vi "RTS Set Chamber Temp Humidity.vi"(5 "Room Setpoints":T7={"Room Setpoint Temperature (*RM Dry Set P1)"=90.0, "Room Setpoint Humidity (*RM Hum Set P1)"=20.0, "Room Cool Temperature (*RM Cool Setp 1)"=65.0, "Room Dehum Temperature (*RM De Hum Set P1)"=60.0} {"Room Dehum Temperature (*RM De Hum Set P1)" min=30.0 max=120.0; "Room Cool Temperature (*RM Cool Setp 1)" min=30.0 max=120.0; "Room Setpoint Humidity (*RM Hum Set P1)" min=5.0 max=98.0; "Room Setpoint Temperature (*RM Dry Set P1)" min=40.0 max=120.0}, 7 "All Door Opener Ctrl":T4 {"Station 8"."Station Slide"."Chamber 1-1"."Start Time" format="%<%X\n%x>T"; "Station 8"."Station Slide"."Chamber 1-1"."End Time" format="%<%X\n%x>T"; "Station 8"."Station Slide"."Time Count (s)" format="%.2f"; "Station 8"."Station Cab"."Chamber 1-1"."Start Time" format="%<%X\n%x>T"; "Station 8"."Station Cab"."Chamber 1-1"."End Time" format="%<%X\n%x>T"; "Station 8"."Station Cab"."Time Count (s)" format="%.2f"; "Station 8"."Station Freezer"."Chamber 1-1"."Start Time" format="%<%X\n%x>T"; "Station 8"."Station Freezer"."Chamber 1-1"."End Time" format="%<%X\n%x>T"; "Station 8"."Station Freezer"."Time Count (s)" format="%.2f"; "Station 7"."Station Slide"."Chamber 1-1"."Start Time" format="%<%X\n%x>T"; "Station 7"."Station Slide"."Chamber 1-1"."End Time" format="%<%X\n%x>T"; "Station 7"."Station Slide"."Time Count (s)" format="%.2f"; "Station 7"."Station Cab"."Chamber 1-1"."Start Time" format="%<%X\n%x>T"; "Station 7"."Station Cab"."Chamber 1-1"."End Time" format="%<%X\n%x>T"; "Station 7"."Station Cab"."Time Count (s)" format="%.2f"; "Station 7"."Station Freezer"."Chamber 1-1"."Start Time" format="%<%X\n%x>T"; "Station 7"."Station Freezer"."Chamber 1-1"."End Time" format="%<%X\n%x>T"; "Station 7"."Station Freezer"."Time Count (s)" format="%.2f"; "Station 6"."Station Slide"."Chamber 1-1"."Start Time" format="%<%X\n%x>T"; "Station 6"."Station Slide"."Chamber 1-1"."End Time" format="%<%X\n%x>T"; "Station 6"."Station Slide"."Time Count (s)" format="%.2f"; "Station 6"."Station Cab"."Chamber 1-1"."Start Time" format="%<%X\n%x>T"; "Station 6"."Station Cab"."Chamber 1-1"."End Time" format="%<%X\n%x>T"; "Station 6"."Station Cab"."Time Count (s)" format="%.2f"; "Station 6"."Station Freezer"."Chamber 1-1"."Start Time" format="%<%X\n%x>T"; "Station 6"."Station Freezer"."Chamber 1-1"."End Time" format="%<%X\n%x>T"; "Station 6"."Station Freezer"."Time Count (s)" format="%.2f"; "Station 5"."Station Slide"."Chamber 1-1"."Start Time" format="%<%X\n%x>T"; "Station 5"."Station Slide"."Chamber 1-1"."End Time" format="%<%X\n%x>T"; "Station 5"."Station Slide"."Time Count (s)" format="%.2f"; "Station 5"."Station Cab"."Chamber 1-1"."Start Time" format="%<%X\n%x>T"; "Station 5"."Station Cab"."Chamber 1-1"."End Time" format="%<%X\n%x>T"; "Station 5"."Station Cab"."Time Count (s)" format="%.2f"; "Station 5"."Station Freezer"."Chamber 1-1"."Start Time" format="%<%X\n%x>T"; "Station 5"."Station Freezer"."Chamber 1-1"."End Time" format="%<%X\n%x>T"; "Station 5"."Station Freezer"."Time Count (s)" format="%.2f"; "Station 4"."Station Slide"."Chamber 1-1"."Start Time" format="%<%X\n%x>T"; "Station 4"."Station Slide"."Chamber 1-1"."End Time" format="%<%X\n%x>T"; "Station 4"."Station Slide"."Time Count (s)" format="%.2f"; "Station 4"."Station Cab"."Chamber 1-1"."Start Time" format="%<%X\n%x>T"; "Station 4"."Station Cab"."Chamber 1-1"."End Time" format="%<%X\n%x>T"; "Station 4"."Station Cab"."Time Count (s)" format="%.2f"; "Station 4"."Station Freezer"."Chamber 1-1"."Start Time" format="%<%X\n%x>T"; "Station 4"."Station Freezer"."Chamber 1-1"."End Time" format="%<%X\n%x>T"; "Station 4"."Station Freezer"."Time Count (s)" format="%.2f"; "Station 3"."Station Slide"."Chamber 1-1"."Start Time" format="%<%X\n%x>T"; "Station 3"."Station Slide"."Chamber 1-1"."End Time" format="%<%X\n%x>T"; "Station 3"."Station Slide"."Time Count (s)" format="%.2f"; "Station 3"."Station Cab"."Chamber 1-1"."Start Time" format="%<%X\n%x>T"; "Station 3"."Station Cab"."Chamber 1-1"."End Time" format="%<%X\n%x>T"; "Station 3"."Station Cab"."Time Count (s)" format="%.2f"; "Station 3"."Station Freezer"."Chamber 1-1"."Start Time" format="%<%X\n%x>T"; "Station 3"."Station Freezer"."Chamber 1-1"."End Time" format="%<%X\n%x>T"; "Station 3"."Station Freezer"."Time Count (s)" format="%.2f"; "Station 2"."Station Slide"."Chamber 1-1"."Start Time" format="%<%X\n%x>T"; "Station 2"."Station Slide"."Chamber 1-1"."End Time" format="%<%X\n%x>T"; "Station 2"."Station Slide"."Time Count (s)" format="%.2f"; "Station 2"."Station Cab"."Chamber 1-1"."Start Time" format="%<%X\n%x>T"; "Station 2"."Station Cab"."Chamber 1-1"."End Time" format="%<%X\n%x>T"; "Station 2"."Station Cab"."Time Count (s)" format="%.2f"; "Station 2"."Station Freezer"."Chamber 1-1"."Start Time" format="%<%X\n%x>T"; "Station 2"."Station Freezer"."Chamber 1-1"."End Time" format="%<%X\n%x>T"; "Station 2"."Station Freezer"."Time Count (s)" format="%.2f"; "Station 1"."Station Slide"."Chamber 1-1"."Start Time" format="%<%X\n%x>T"; "Station 1"."Station Slide"."Chamber 1-1"."End Time" format="%<%X\n%x>T"; "Station 1"."Station Slide"."Time Count (s)" format="%.2f"; "Station 1"."Station Cab"."Chamber 1-1"."Start Time" format="%<%X\n%x>T"; "Station 1"."Station Cab"."Chamber 1-1"."End Time" format="%<%X\n%x>T"; "Station 1"."Station Cab"."Time Count (s)" format="%.2f"; "Station 1"."Station Freezer"."Chamber 1-1"."Start Time" format="%<%X\n%x>T"; "Station 1"."Station Freezer"."Chamber 1-1"."End Time" format="%<%X\n%x>T"; "Station 1"."Station Freezer"."Time Count (s)" format="%.2f"}, 8 "Error In":errorcluster, 11 "Modbus Master in":refnum<class "Modbus Master.lvclass">) -> (0 "Error Out":errorcluster, 1 "Matching Setpoints?":bool, 2 "Set Chamber Conditions":bool, 3 "Modbus master out":refnum<class "Modbus Master.lvclass">, 4 "Chamber 1-1":T1 {"Start Time" format="%<%X\n%x>T"; "End Time" format="%<%X\n%x>T"}, 6 "Index":i32)   [LabVIEW 2016]
uses:
  Type Definitions/RTS Chamber Temperature Humidity Control.ctl
  <vilib>/NI/Modbus Library/API/Master/Modbus Master.lvclass
  Type Definitions/RTS All Station Door Opener Ctrl.ctl
  Type Definitions/RTS Station Relay Ops.ctl
  Type Definitions/RTS Door Opener Indicator.ctl
  Type Definitions/RTS Door Ops Client.ctl
  Type Definitions/RTS Door Opening Schedule.ctl
  Type Definitions/RTS Door Ops Sequence.ctl
panel:
  # "Chamber Conditions:"
  # "Chamber Conditions:"
  # "Chamber Conditions:"
  # "Chamber Conditions:"
  # "Chamber Conditions:"
  # "Chamber Conditions:"
  # "Chamber Conditions:"
  # "Chamber Conditions:"
  # "Chamber Conditions:"
  # "Chamber Conditions:"
  # "Chamber Conditions:"
  # "Chamber Conditions:"
  # "Chamber Conditions:"
  # "Chamber Conditions:"
  # "Chamber Conditions:"
  # "Chamber Conditions:"
  # "Chamber Conditions:"
  # "Chamber Conditions:"
  # "Chamber Conditions:"
  # "Chamber Conditions:"
  # "Chamber Conditions:"
  # "Chamber Conditions:"
  # "Chamber Conditions:"
  # "Chamber Conditions:"
  # "Chamber Conditions:"
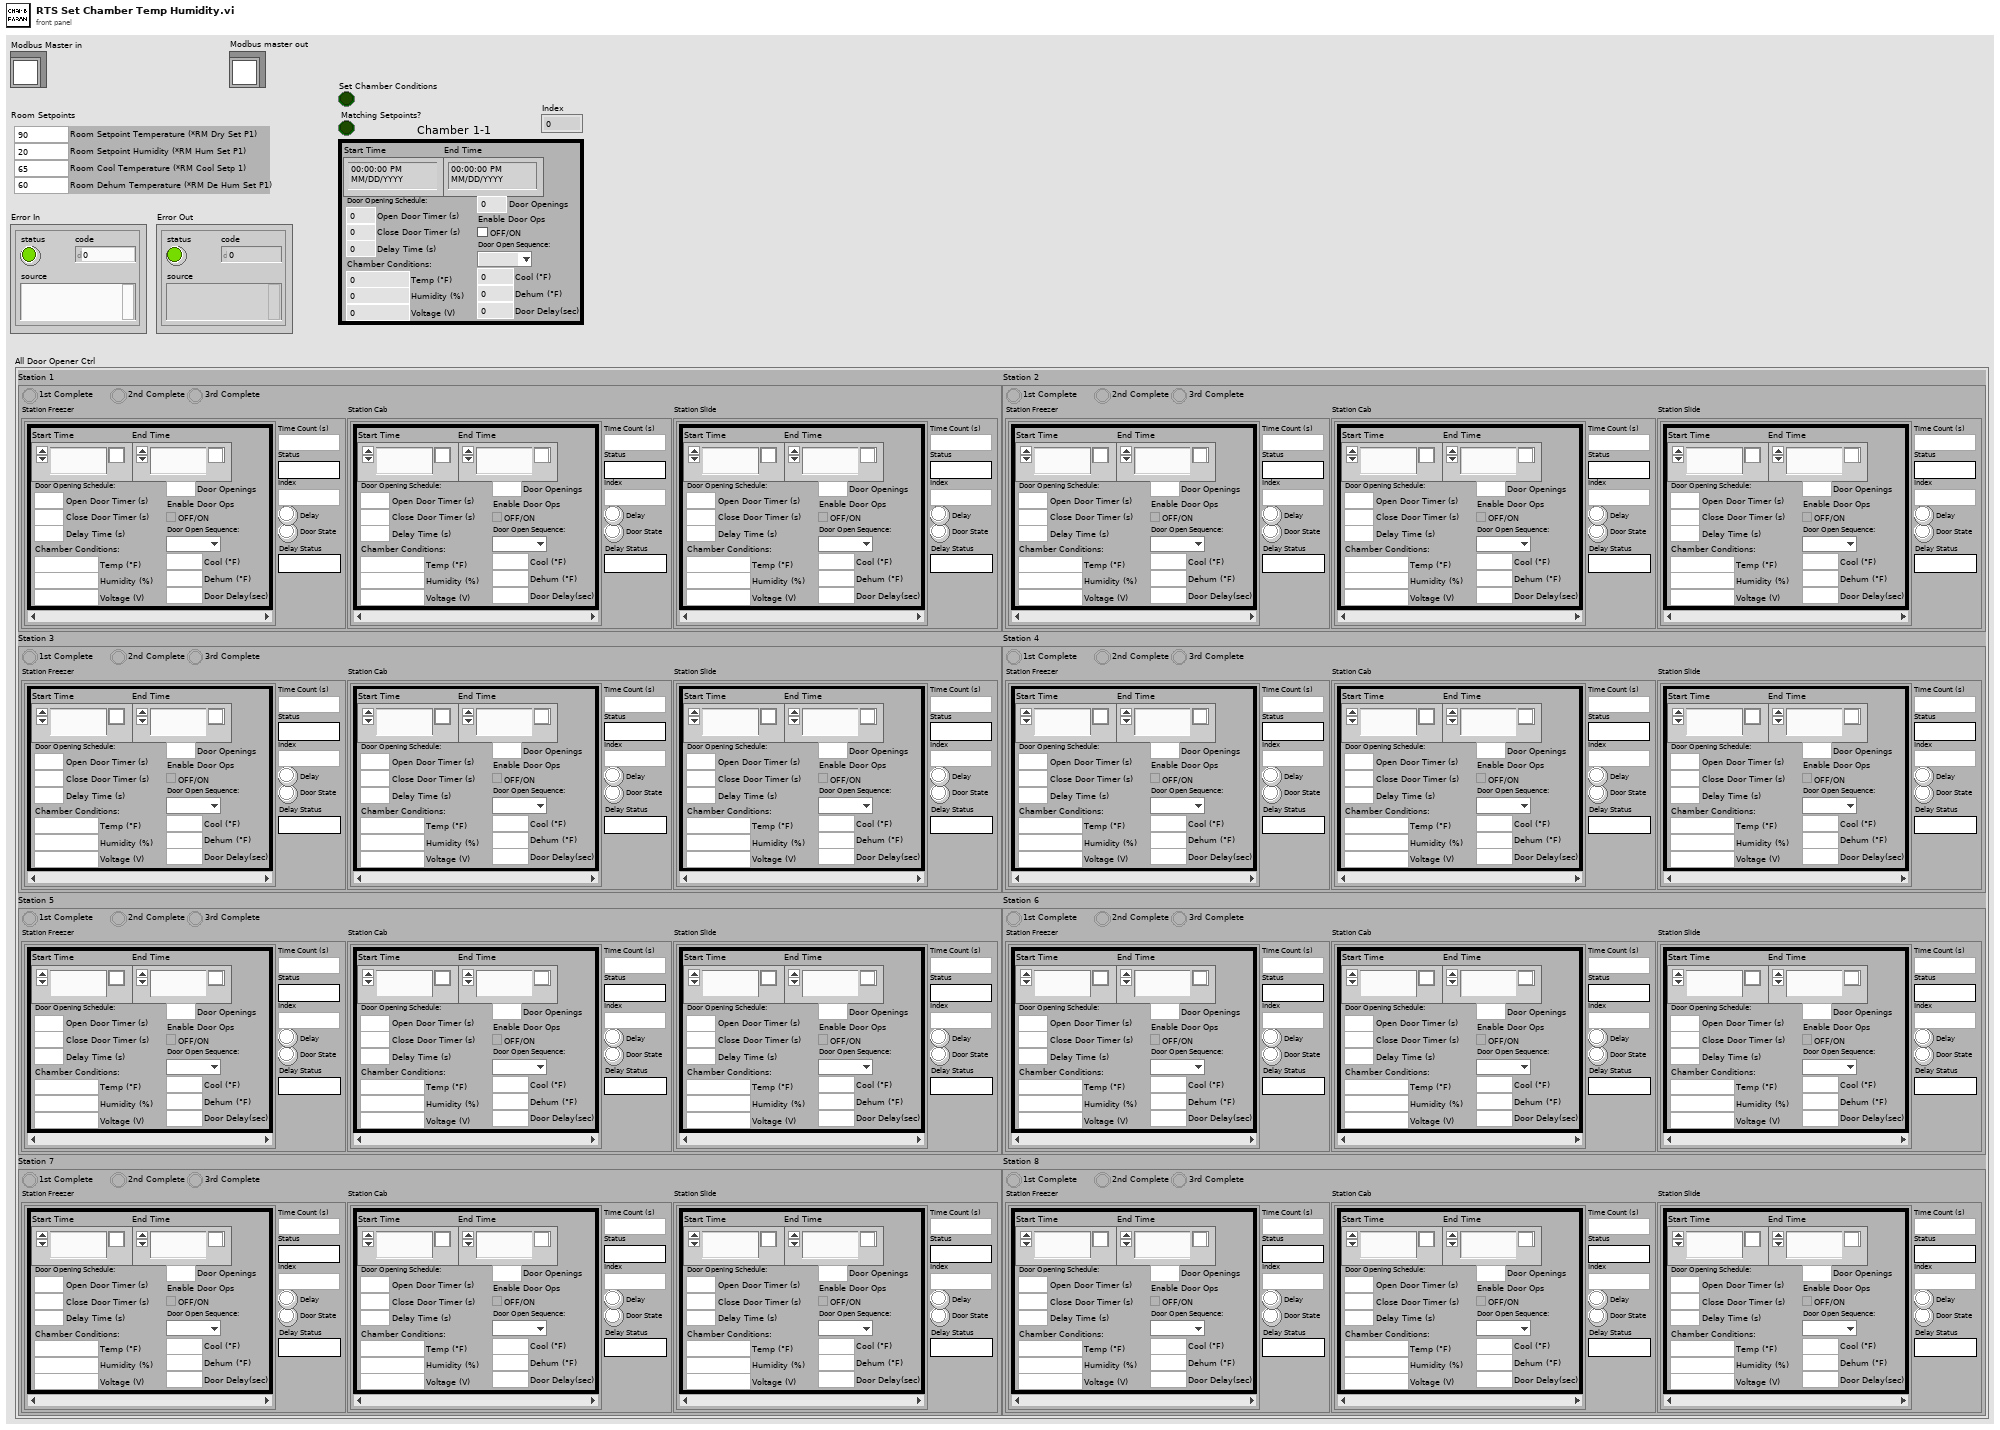
[diagram p1: front panel]
types:
  T1 = typedef "RTS Door Ops Client.ctl" = cluster{"End Time":timestamp, "Start Time":timestamp, "Door Opening Schedule:":T2, "Enable Door Ops":bool, "Door Openings":u32, "Temp (°F)":dbl, "Humidity (%)":dbl, "Voltage (V)":dbl, "Door Open Sequence:":T3, "Door Delay(sec)":dbl, "Dehum (°F)":dbl, "Cool (°F)":dbl}
  T2 = typedef "RTS Door Opening Schedule.ctl" = cluster{"Open Door Timer (s)":dbl, "Delay Time (s)":dbl, "Close Door Timer (s)":dbl}
  T3 = typedef "RTS Door Ops Sequence.ctl" = enum16{"", "1st", "2nd", "3rd"}
  T4 = typedef "RTS All Station Door Opener Ctrl.ctl" = cluster{"Station 1":T5, "Station 2":T5, "Station 3":T5, "Station 4":T5, "Station 5":T5, "Station 6":T5, "Station 7":T5, "Station 8":T5}
  T5 = typedef "RTS Station Relay Ops.ctl" = cluster{"Station Freezer":T6, "Station Cab":T6, "Station Slide":T6, "1st Complete":bool, "2nd Complete":bool, "3rd Complete":bool}
  T6 = typedef "RTS Door Opener Indicator.ctl" = cluster{"Time Count (s)":dbl, "Status":string, "Door State":bool, "Delay":bool, "Chamber 1-1":T1[], "Index":i32, "Delay Status":string}
  T7 = typedef "RTS Chamber Temperature Humidity Control.ctl" = cluster{"Room Setpoint Temperature (*RM Dry Set P1)":dbl, "Room Setpoint Humidity (*RM Hum Set P1)":dbl, "Room Cool Temperature (*RM Cool Setp 1)":dbl, "Room Dehum Temperature (*RM De Hum Set P1)":dbl}
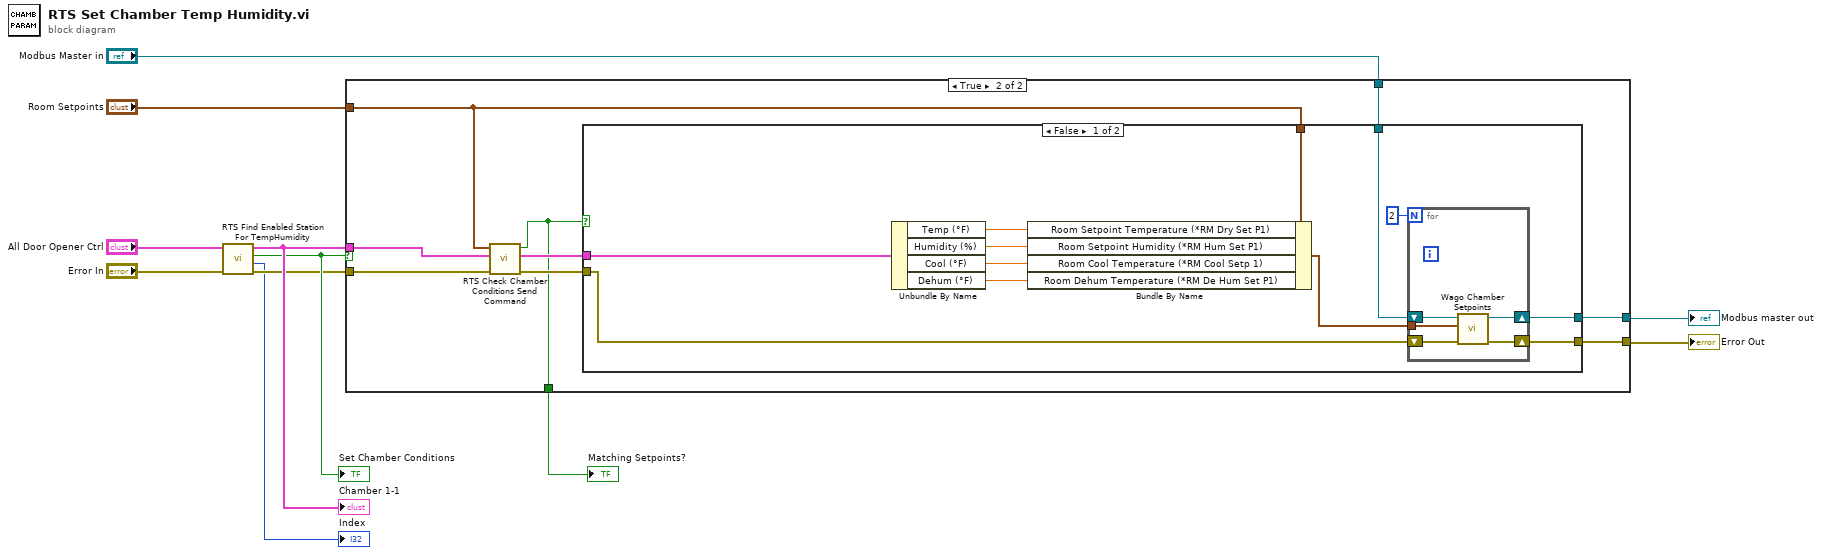
[diagram p0: block diagram]
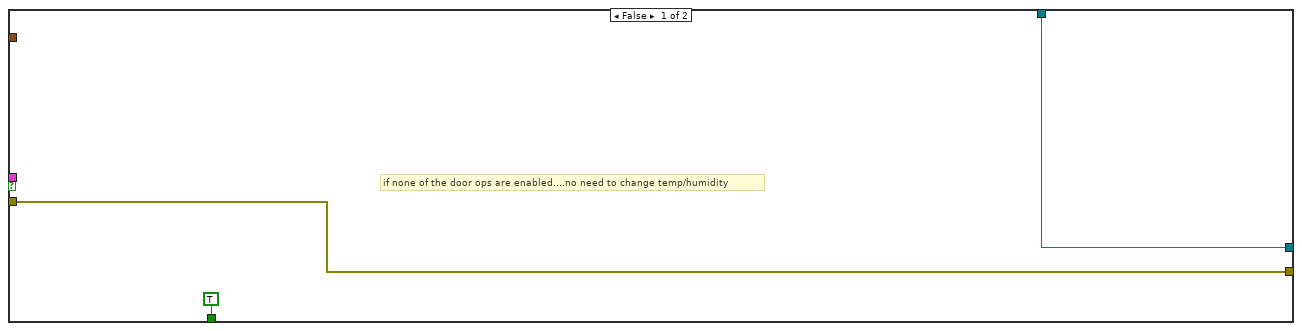
[diagram p2: hidden frame]
diagram:
  n1 = call "RTS Find Enabled Station For TempHumidity.vi"("Error In"="Error In", "All Door Opener Ctrl"="All Door Opener Ctrl") -> ("Error Out"=w3:errorcluster, "Index"=→"Index":i32, "Set Chamber Conditions"=w5:bool, "Chamber 1-1"=w7:T1)  [unwired: 6 in]
  "Set Chamber Conditions" <- w5
  "Chamber 1-1" <- w7
  n2 = case shown="True" w5 {
    tunnel: [w13 w23] -> w11
    tunnel: "Modbus Master in" -> [w14 w22]
    tunnel: [w14 w21] -> w9
    tunnel: w7 -> [_ w20]
    tunnel: "Room Setpoints" -> [_ w16]
    tunnel: w3 -> [w13 w18]
    tunnel: [TRUE ("Matching Setpoints?") w15] -> w2
    frame False {
      # "if none of the door ops are enabled....no need to change temp/humidity"
    }
    frame True {
      n3 = call "RTS Check Chamber Conditions Send Command.vi"("Error In"=w18, "Chamber 1-1"=w20, "Room Setpoints"=w16) -> ("Error Out"=w17:errorcluster, "New Conditions"=w19:T1, "Matching Setpoints?"=w15:bool)  [unwired: 6 in]
      n4 = case shown="False" w15 {
        tunnel: [w35 w41] -> w23
        tunnel: w22 -> [w34 w42]
        tunnel: [w33 w42] -> w21
        tunnel: w16 -> [w32 _]
        tunnel: w19 -> [w29 _]
        tunnel: w17 -> [w30 w41]
        frame False {
          n5 = Unbundle By Name(w29) -> ("Temp (°F)"=w28:dbl, "Humidity (%)"=w27:dbl, "Cool (°F)"=w26:dbl, "Dehum (°F)"=w25:dbl)
          n6 = Bundle By Name(cluster=w32, "Room Setpoint Temperature (*RM Dry Set P1)"=w28, "Room Setpoint Humidity (*RM Hum Set P1)"=w27, "Room Cool Temperature (*RM Cool Setp 1)"=w26, "Room Dehum Temperature (*RM De Hum Set P1)"=w25) -> (w31:T7)
          n7 = for {
            N: 2 -> [_]
            tunnel: w31 -> [w37]
            shift-right: [w38] -> w33
            shift-left: w34 -> [w39]
            shift-right: [w40] -> w35
            shift-left: w30 -> [w36]
            n8 = call "Wago Chamber Setpoints.vi"("error in (no error)"=w36, "Room Setpoints"=w37, "Modbus Master in"=w39) -> ("error out"=w40:errorcluster, "Modbus master out"=w38:refnum<class "Modbus Master.lvclass">)  [unwired: 7 in]
          }
        }
        frame True {
        }
      }
    }
  }
  "Error Out" <- w11
  "Modbus master out" <- w9
  "Matching Setpoints?" <- w2
